vi "test Boolean.vi"(8 "error in (no error)":errorcluster, 11 "TestCase in":refnum<class "Scan From Python String Tests.lvclass">) -> (0 "error out":errorcluster, 3 "TestCase out":refnum<class "Scan From Python String Tests.lvclass">)   [LabVIEW 2020, in "Scan From Python String Tests.lvclass"]
uses:
  Scan From Python String Tests.lvclass
  source/Python String to LabVIEW Data/Python String to LabVIEW Data (Boolean).vi
  Scan From Python String Tests.lvclass/Scan From Python String Tests.ctl
  <vilib>/addons/_JKI Toolkits/VI Tester/TestCase.llb/TestCase.lvclass
  source/jki_python_data_tools.lvlib
  C:/Program Files/National Instruments/LabVIEW 2020/vi.lib/addons/_JKI Toolkits/VI Tester/TestCase.llb/TestCase.lvclass
panel:
  out "Failures":T1(array[cluster])
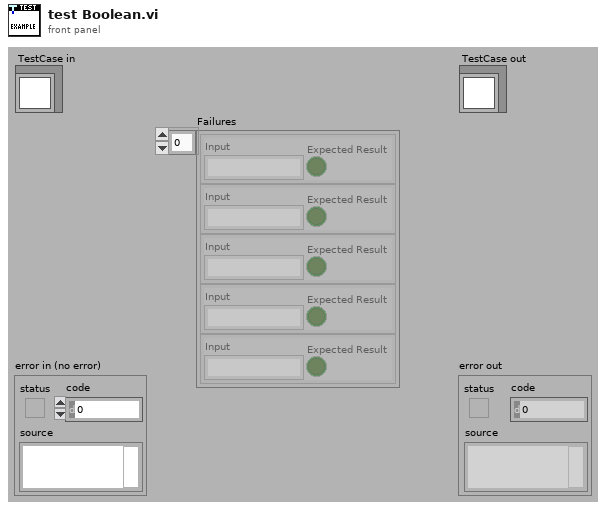
[diagram p1: front panel]
types:
  T1 = cluster{"Input":string, "Expected Result":bool}[]
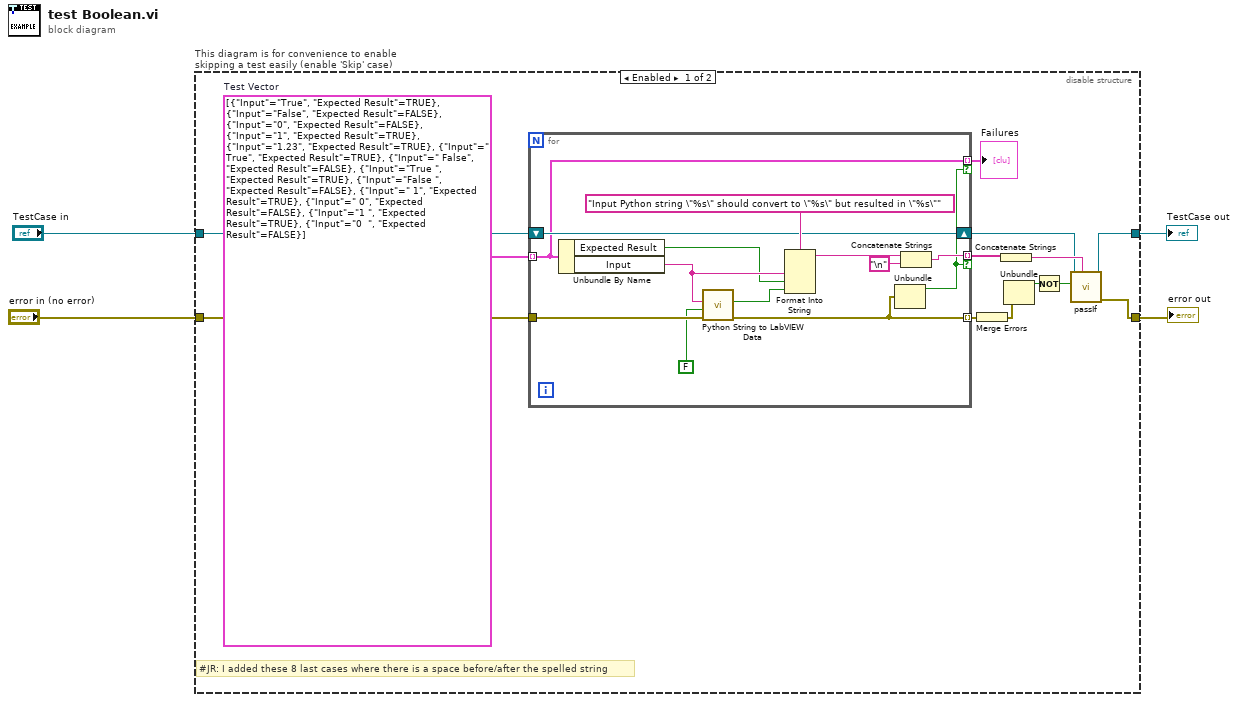
[diagram p0: block diagram]
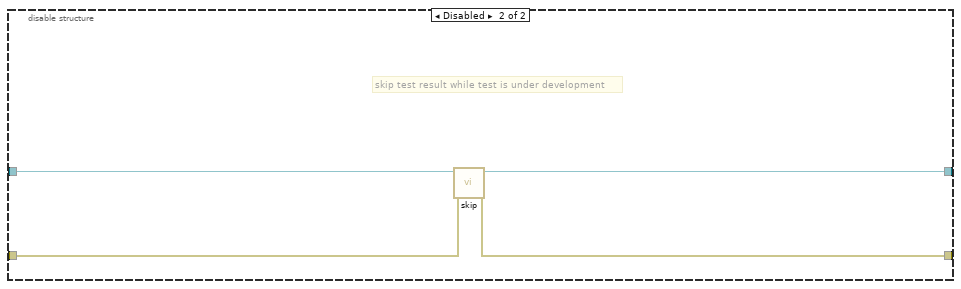
[diagram p2: hidden frame]
diagram:
  n1 = disable-structure "This diagram is for convenience to enable skipping a test easily (enable 'Skip' case)" shown="Enabled" {
    disable-tunnel: "TestCase in" -> [w15 w34]
    disable-tunnel: [w6 w32] -> w1
    disable-tunnel: [w8 w33] -> w3
    disable-tunnel: "error in (no error)" -> [w17 w31]
    frame Enabled {
      w16 = T1 [{"Input"="True", "Expected Result"=TRUE}, {"Input"="False", "Expected Result"=FALSE}, {"Input"="0", "Expected Result"=FALSE}, {"Input"="1", "Expected Result"=TRUE}, {"Input"="1.23", "Expected Result"=TRUE}, {"Input"=" True", "Expected Result"=TRUE}, {"Input"=" False", "Expected Result"=FALSE}, {"Input"="True ", "Expected Result"=TRUE}, {"Input"="False ", "Expected Result"=FALSE}, {"Input"=" 1", "Expected Result"=TRUE}, {"Input"=" 0", "Expected Result"=FALSE}, {"Input"="1 ", "Expected Result"=TRUE}, {"Input"="0  ", "Expected Result"=FALSE}]  # Test Vector
      # "#JR: I added these 8 last cases where there is a space before/after the spelled string"
      n2 = for {
        tunnel: w16 -> [w19] mode=indexing
        shift-right: [w24] -> w7
        shift-left: w15 -> [w24]
        tunnel: w17 -> [w30]
        tunnel: [w23] -> w13 mode=indexing
        tunnel: [w20] -> w14 mode=indexing if=w18
        tunnel: [w19] -> w5 mode=indexing if=w18
        n3 = Unbundle By Name(w19) -> ("Expected Result"=w25:bool, "Input"=w29:string)
        n4 = call-poly "Python String to LabVIEW Data.vi"("error in (no error)"=w30, "type"=FALSE ("Default Value"), "Python String"=w29) -> ("error out"=w23:errorcluster, "LabVIEW Data"=w28:bool)  [unwired: 7 in]
        n5 = Format Into String(format string="Input Python string \"%s\" should convert to \"%s\" but resulted in \"%s\"", w29, w25, w28) -> (resulting string=w21:string)  [unwired: 2 in, 1 out]
        n6 = Unbundle(w23) -> ("status"=w18:bool)  [unwired: 2 out]
        n7 = Concatenate Strings(w21, "\n") -> (w20:string)
      }
      "Failures" <- w5
      n8 = Merge Errors(w13) -> (w10:errorcluster)
      n9 = Concatenate Strings(w14) -> (w12:string)
      n10 = Unbundle(w10) -> ("status"=w11:bool)  [unwired: 2 out]
      n11 = Not(x=w11) -> (.not. x?=w9:bool)
      n12 = call-dynamic "passIf.vi"("custom report message (\"\")"=w12, "pass"=w9, "TestCase in"=w7) -> ("error out"=w8:errorcluster, "TestCase out"=w6:refnum<class "Scan From Python String Tests.lvclass">)  [unwired: 7 in]
    }
    frame Disabled {
      # "skip test result while test is under development"
      n13 = call <vilib>:"skip.vi"("error in (no error)"=w31, "TestCase in"=w34) -> ("error out"=w33:errorcluster, "TestCase out"=w32:refnum<class "Scan From Python String Tests.lvclass">)  [unwired: 8 in]
    }
  }
  "error out" <- w3
  "TestCase out" <- w1
